vi "Add RS485 Address.vi"(4 "error in":errorcluster, 6 "Command (input)":string, 7 "VISA resource name in":refnum<visa-resource-name>) -> (0 "error out":errorcluster, 2 "Command (output)":string, 3 "VISA resource name out":refnum<visa-resource-name>)   [LabVIEW 2018, in "JULABO DeviceDriver.lvlib"]
uses:
  JULABO DeviceDriver.lvlib
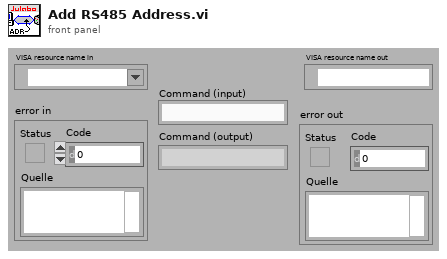
[diagram p1: front panel]
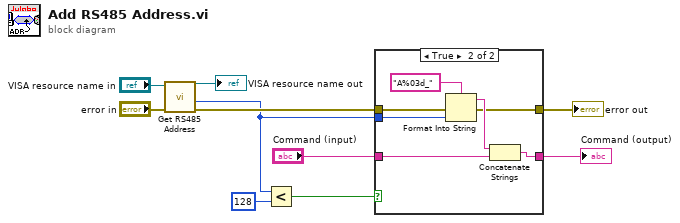
[diagram p0: block diagram]
diagram:
  n1 = call "Get RS485 Address.vi"("error in"="error in", "VISA resource name in"="VISA resource name in") -> ("Fehler (Ausgang)"=w4:errorcluster, "RS485-Address"=w1:u8, "VISA resource name out"=→"VISA resource name out":refnum<visa-resource-name>)  [unwired: 3 in]
  n2 = Less?(x=w1, y=u32 128) -> (x < y?=w8:bool)
  n3 = case shown="True" w8 {
    tunnel: [w12 w16] -> w6
    tunnel: "Command (input)" -> [w12 w14]
    tunnel: w4 -> [w11 w19]
    tunnel: w1 -> [_ w18]
    tunnel: [w11 w13] -> w3
    frame False {
    }
    frame True {
      n4 = Format Into String(format string="A%03d_" ("Format-String"), error in=w19, w18) -> (resulting string=w15:string, error out=w13:errorcluster)  [unwired: 1 in]
      n5 = Concatenate Strings(w15, w14) -> (w16:string)
    }
  }
  "error out" <- w3
  "Command (output)" <- w6
